vi "读取产品参数信息-CCD6.vi"(8 "错误输入（无错误）":errorcluster, 11 "LoadProductName":string) -> (0 "错误输出":errorcluster)   [LabVIEW 2017]
uses:
  Global System.vi
panel:
  out "添加的路径":path
  out "连接的字符串":string
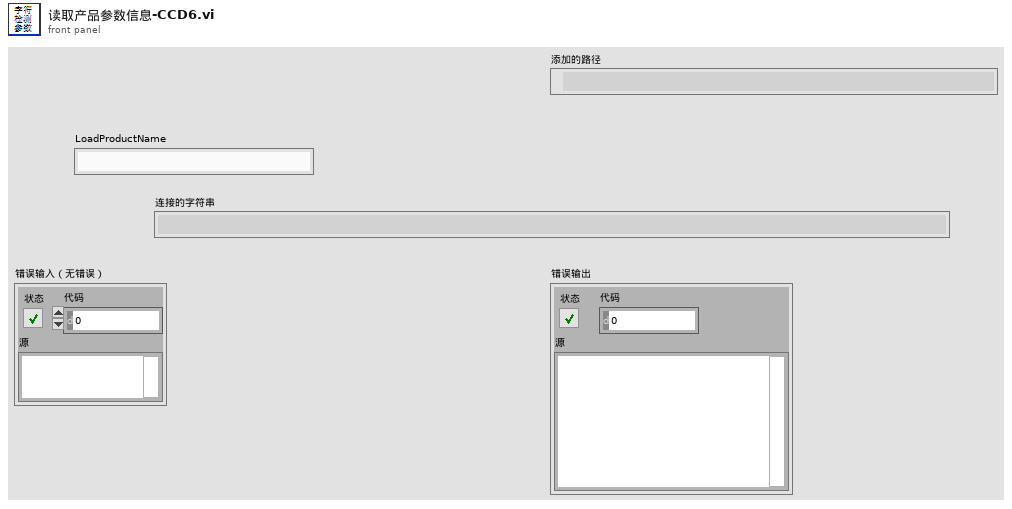
[diagram p1: front panel]
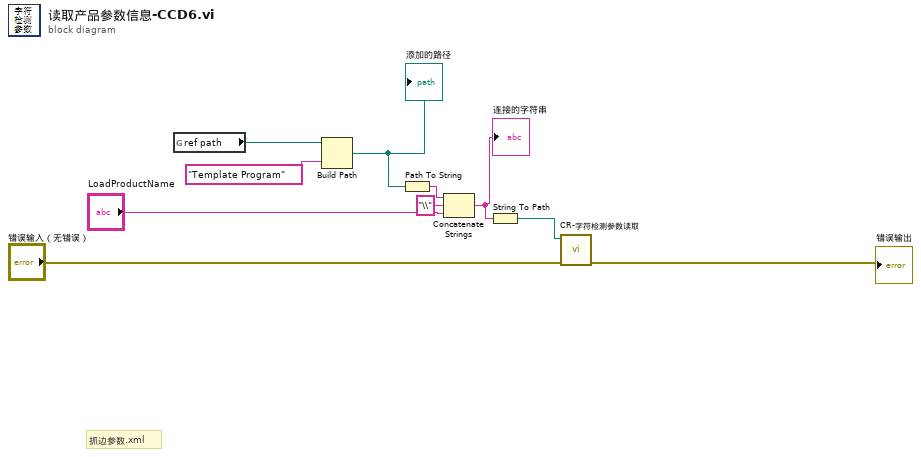
[diagram p0: block diagram]
diagram:
  # "抓边参数.xml"
  n1 = global read "Global System.vi" "ref path"() -> (w10:path)
  n2 = Build Path(base path=w10, name or relative path="Template Program" ("名称或相对路径")) -> (appended path=w8:path)
  "添加的路径" <- w8
  n3 = Path To String(path=w8) -> (string=w7:string)
  n4 = Concatenate Strings(w7, "\\" ("字符串"), "LoadProductName") -> (w4:string)
  "连接的字符串" <- w4
  n5 = String To Path(string=w4) -> (path=w3:path)
  n6 = call "CR-字符检测参数读取.vi"("error in (no error)"="错误输入（无错误）", "基路径"=w3) -> ("error out"=→"错误输出":errorcluster)  [unwired: 5 in, 3 out]
